vi "CalcWinBounds.vi"(7 "Mouse device ID":refnum<k1>, 9 "WindowSize":cluster{"Width":i32, "Height":i32}={"Width"=268, "Height"=320}) -> (3 "Window Bounds":T1)   [LabVIEW 2016]
uses:
  <vilib>/Utility/miscctls.llb/LVRectTypeDef.ctl
  <vilib>/Utility/inputDevices.llb/mouseAcquire.vi
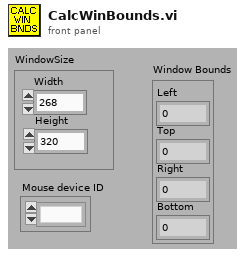
[diagram p1: front panel]
types:
  T1 = typedef "LVRectTypeDef.ctl" = cluster{"Left":i16, "Top":i16, "Right":i16, "Bottom":i16}
  T2 = cluster{"Horizontal":i32, "Vertical":i32, "Scrolling":i32}
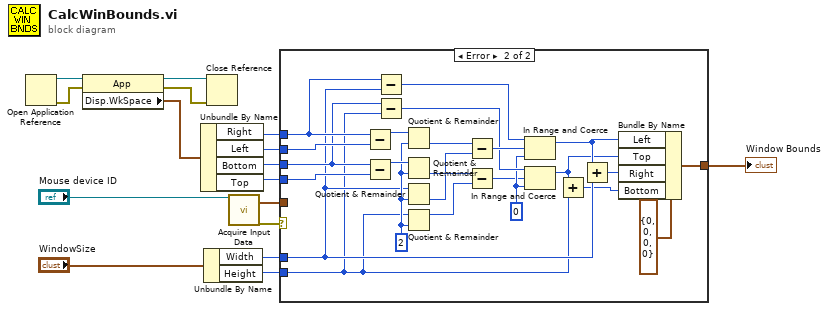
[diagram p0: block diagram]
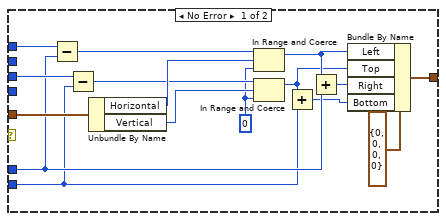
[diagram p2: hidden frame]
diagram:
  n1 = Open Application Reference() -> (0:w13:errorcluster, 3:w16:refnum<vi>)  [unwired: 1 in, 3 out]
  n2 = property class="App"(reference=w16, error in=w13) -> (reference out=w15:refnum<vi>, error out=w14:errorcluster, "Disp.WkSpace"=w9:T1)
  n3 = Unbundle By Name(w9) -> ("Right"=w8:i16, "Left"=w7:i16, "Bottom"=w6:i16, "Top"=w5:i16)
  n4 = Unbundle By Name("WindowSize") -> ("Width"=w2:i32, "Height"=w1:i32)
  n5 = Close Reference(reference=w15, error in (no error)=w14) -> ()  [unwired: 1 out]
  n6 = call-poly <vilib>:"Acquire Input Data.vi"("device ID"="Mouse device ID") -> ("axis info"=w12:T2, "error out"=w11:errorcluster)  [unwired: 2 in, 15 out]
  n7 = case shown="Error" w11 {
    tunnel: w12 -> [w30 _]
    tunnel: w8 -> [w32 w48]
    tunnel: w7 -> [_ w52]
    tunnel: w6 -> [w31 w46]
    tunnel: w5 -> [_ w51]
    tunnel: w2 -> [w24 w40]
    tunnel: w1 -> [w23 w39]
    tunnel: [w17 w34] -> w4
    frame No Error {
      w25 = 0 ("lower limit")
      n8 = Subtract(x=w32, y=w24) -> (x-y=w29:i32)
      n9 = Subtract(x=w31, y=w23) -> (x-y=w27:i32)
      n10 = Unbundle By Name(w30) -> ("Horizontal"=w28:i32, "Vertical"=w26:i32)
      n11 = In Range and Coerce(upper limit=w29, x=w28, lower limit=w25) -> (coerced(x)=w22:i32)  [unwired: 1 out]
      n12 = In Range and Coerce(upper limit=w27, x=w26, lower limit=w25) -> (coerced(x)=w21:i32)  [unwired: 1 out]
      n13 = Add(x=w21, y=w23) -> (x+y=w19:i32)
      n14 = Add(x=w22, y=w24) -> (x+y=w20:i32)
      n15 = Bundle By Name(cluster=T1 {"Left"=0, "Top"=0, "Right"=0, "Bottom"=0} ("Front Panel Window:Window Bounds"), "Left"=w22, "Top"=w21, "Right"=w20, "Bottom"=w19) -> (w17:T1)
    }
    frame Error {
      w47 = i16 2 ("y")
      w42 = 0 ("lower limit")
      n16 = Subtract(x=w48, y=w52) -> (x-y=w56:i16)
      n17 = Subtract(x=w46, y=w51) -> (x-y=w55:i16)
      n18 = Subtract(x=w48, y=w40) -> (x-y=w45:i32)
      n19 = Subtract(x=w46, y=w39) -> (x-y=w43:i32)
      n20 = Quotient & Remainder(x=w56, y=w47) -> (floor(x/y)=w54:i16)  [unwired: 1 out]
      n21 = Quotient & Remainder(x=w55, y=w47) -> (floor(x/y)=w53:i16)  [unwired: 1 out]
      n22 = Quotient & Remainder(x=w40, y=w47) -> (floor(x/y)=w50:i32)  [unwired: 1 out]
      n23 = Quotient & Remainder(x=w39, y=w47) -> (x-y*floor(x/y)=w49:i32)  [unwired: 1 out]
      n24 = Subtract(x=w54, y=w50) -> (x-y=w44:i32)
      n25 = Subtract(x=w53, y=w49) -> (x-y=w41:i32)
      n26 = In Range and Coerce(upper limit=w45, x=w44, lower limit=w42) -> (coerced(x)=w38:i32)  [unwired: 1 out]
      n27 = In Range and Coerce(upper limit=w43, x=w41, lower limit=w42) -> (coerced(x)=w36:i32)  [unwired: 1 out]
      n28 = Add(x=w36, y=w39) -> (x+y=w35:i32)
      n29 = Add(x=w38, y=w40) -> (x+y=w37:i32)
      n30 = Bundle By Name(cluster=T1 {"Left"=0, "Top"=0, "Right"=0, "Bottom"=0} ("Front Panel Window:Window Bounds"), "Left"=w38, "Top"=w36, "Right"=w37, "Bottom"=w35) -> (w34:T1)
    }
  }
  "Window Bounds" <- w4
